vi "PCO_SetFanControlParameters.vi"(8 "error in (no error)":errorcluster {"code" format="%x"}, 9 "wValue":u16, 10 "wMode":u16, 11 "ph":u64) -> (0 "error out":errorcluster {"code" format="%x"}, 2 "ErrorMessage":i32 format="%x", 3 "ph out":u64)   [LabVIEW 2019, in "SDK.lvlib" / "GeneralCameraControl.lvlib"]
doc: "SC2_SDK_FUNC int WINAPI PCO_SetFanControlParameters(HANDLE hCam, WORD wMode, WORD wValue, WORD wReserved);"
uses:
  GeneralCameraControl.lvlib
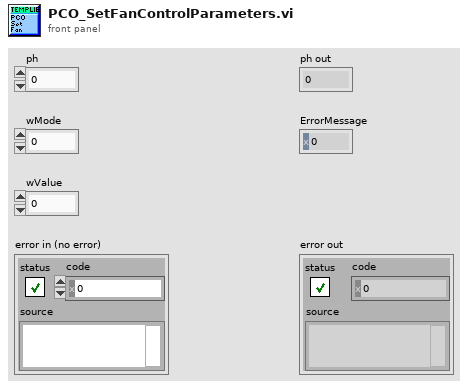
[diagram p1: front panel]
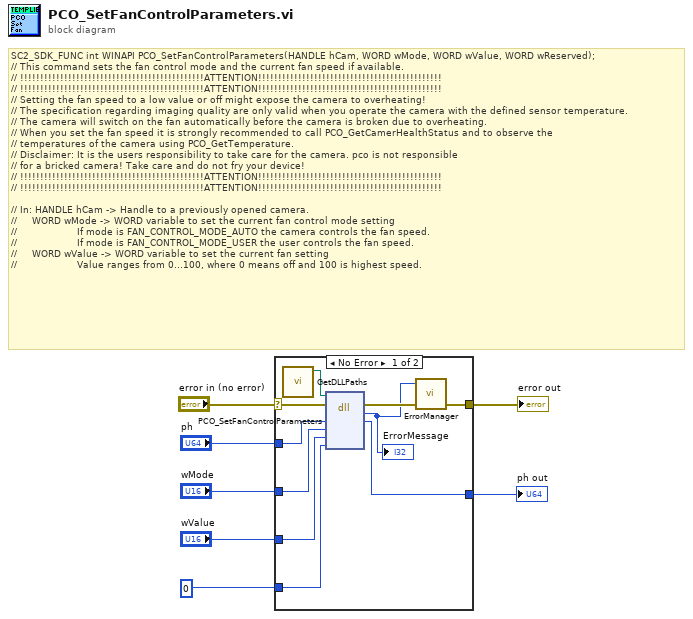
[diagram p0: block diagram]
diagram:
  # "SC2_SDK_FUNC int WINAPI PCO_SetFanControlParameters(HANDLE hCam, WORD wMode, WORD wValue, WORD wReserved);\n// This command sets the fan control mode and the current fan speed if available.\n// !!!!!!!!!!!!!!!!!!!!!!!!!!!!!!!!!!!!!!!!!!!!!!ATTENTION!!!!!!!!!!!!!!!!!!!!!!!!!!!!!!!!!!!!!!!!!!!!!!\n// !!!!!!!!!!!!!!!!!!!!!!!!!!!!!!!!!!!!!!!!!!!!!!ATTENTION!!!!!!!!!!!!!!!!!!!!!!!!!!!!!!!!!!!!!!!!!!!!!!\n// Setting the fan speed to a low value or off might expose the camera to overheating!\n// The specification regarding imaging quality are only valid when you operate the camera with the defined sensor temperature.\n// The camera will switch on the fan automatically before the camera is broken due to overheating.\n// When you set the fan speed it is strongly recommended to call PCO_GetCamerHealthStatus and to observe the\n// temperatures of the camera using PCO_GetTemperature.\n// Disclaimer: It is the users responsibility to take care for the camera. pco is not responsible \n// for a bricked camera! Take care and do not fry your device!\n// !!!!!!!!!!!!!!!!!!!!!!!!!!!!!!!!!!!!!!!!!!!!!!ATTENTION!!!!!!!!!!!!!!!!!!!!!!!!!!!!!!!!!!!!!!!!!!!!!!\n// !!!!!!!!!!!!!!!!!!!!!!!!!!!!!!!!!!!!!!!!!!!!!!ATTENTION!!!!!!!!!!!!!!!!!!!!!!!!!!!!!!!!!!!!!!!!!!!!!!\n\n// In: HANDLE hCam -> Handle to a previously opened camera.\n//     WORD wMode -> WORD variable to set the current fan control mode setting\n//                    If mode is FAN_CONTROL_MODE_AUTO the camera controls the fan speed.\n//                    If mode is FAN_CONTROL_MODE_USER the user controls the fan speed.\n//     WORD wValue -> WORD variable to set the current fan setting\n//                    Value ranges from 0...100, where 0 means off and 100 is highest speed."
  n1 = case shown="No Error" "error in (no error)" {
    selector: "error in (no error)" -> [w12 w19]
    tunnel: "ph" -> [w17 w18]
    tunnel: [w16 w18] -> w6
    tunnel: "wMode" -> [w15 _]
    tunnel: "wValue" -> [w14 _]
    tunnel: [w10 w19] -> w3
    tunnel: u16 0 ("wReserved") -> [w13 _]
    frame No Error {
      n2 = call "GetDLLPaths.vi"() -> ("SC2_Cam_Path"=w8:path)  [unwired: 9 in, 2 out]
      n3 = dll-call lib="?" fn="PCO_SetFanControlParameters"(path in=w8, error in=w12, "ph"=w17, "wMode"=w15, "wValue"=w14, "wReserved"=w13) -> (error out=w11:errorcluster, "return type"=w9:i32, "ph"=w16:u64)  [unwired: 4 in, 1 out]
      "ErrorMessage" <- w9
      n4 = call "ErrorManager.vi"("error in (no error)"=w11, "error code"=w9) -> ("error out"=w10:errorcluster)  [unwired: 3 in]
    }
    frame Error {
    }
  }
  "ph out" <- w6
  "error out" <- w3
